vi "Get Build Version.vi"(8 "error in":errorcluster caption="Error In", 10 "Build Spec Name":string, 11 "Project Path":path) -> (0 "error out":errorcluster caption="Error Out", 3 "Version":string)   [LabVIEW 2015]
doc: "Open the VI reference pointed by the VI Name input. This function does not require a path as input but requires that the VI is present in the same project as the calling VI."
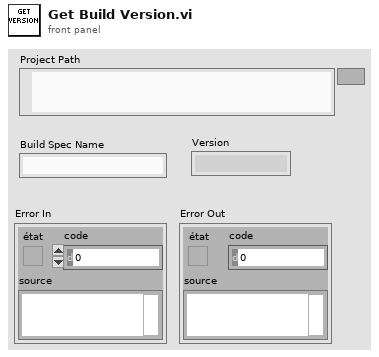
[diagram p1: front panel]
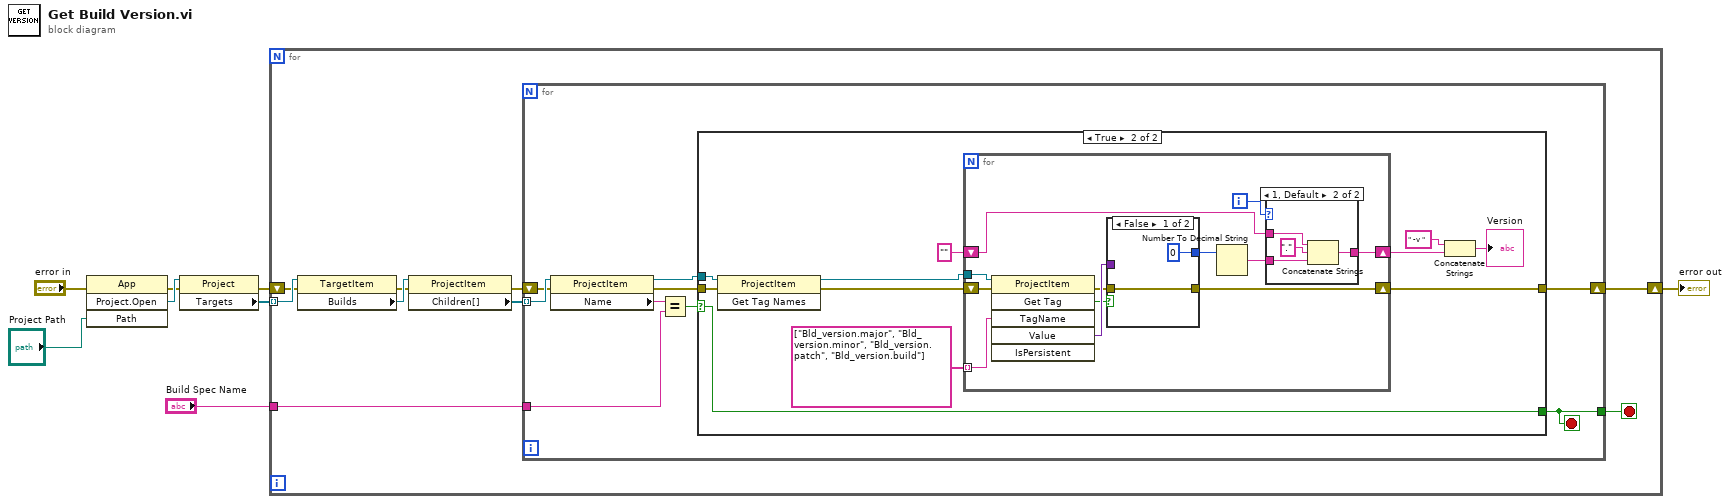
[diagram p0: block diagram]
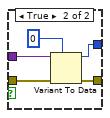
[diagram p4: hidden frame]
diagram:
  n1 = invoke class="App" method="Project.Open"(error in="error in", "Path"="Project Path") -> (error out=w4:errorcluster, "Project:Open"=w5:refnum<vi>)  [unwired: 2 in, 2 out]
  n2 = property class="Project"(reference=w5, error in=w4) -> (error out=w2:errorcluster, "Targets"=w8:refnum<vi>[])  [unwired: 1 out]
  n3 = for {
    tunnel: w8 -> [w17] mode=indexing
    tunnel: "Build Spec Name" -> [w14]
    shift-right: [w9] -> w1
    shift-left: w2 -> [w10]
    stop <- w12 stop-if-true
    n4 = property class="TargetItem"(reference=w17, error in=w10) -> (error out=w13:errorcluster, "Builds"=w16:refnum<vi>)  [unwired: 1 out]
    n5 = property class="ProjectItem"(reference=w16, error in=w13) -> (error out=w11:errorcluster, "Children[]"=w15:refnum<vi>[])  [unwired: 1 out]
    n6 = for {
      tunnel: w15 -> [w24] mode=indexing
      tunnel: w14 -> [w25]
      tunnel: [w22] -> w12
      shift-right: [w18] -> w9
      shift-left: w11 -> [w21]
      stop <- w22 stop-if-true
      n7 = property class="ProjectItem"(reference=w24, error in=w21) -> (reference out=w19:refnum<vi>, error out=w20:errorcluster, "Name"=w26:string)
      n8 = Equal?(x=w26, y=w25) -> (x = y?=w23:bool)
      n9 = case shown="True" w23 {
        selector: w23 -> [_ w37]
        tunnel: w19 -> [_ w38]
        tunnel: [_ w37] -> w22
        tunnel: w20 -> [w27 w33]
        tunnel: [w27 w31] -> w18
        frame False {
        }
        frame True {
          n10 = invoke class="ProjectItem" method="Get Tag Names"(reference=w38, error in=w33) -> (reference out=w36:refnum<vi>, error out=w32:errorcluster)  [unwired: 1 in, 1 out]
          n11 = for {
            tunnel: w36 -> [w49]
            tunnel: string[] ["Bld_version.major", "Bld_version.minor", "Bld_version.patch", "Bld_version.build"] -> [w48] mode=indexing
            shift-right: [w43] -> w29
            shift-left: "" -> [w44]
            shift-right: [w39] -> w31
            shift-left: w32 -> [w41]
            i -> [w42]
            n12 = invoke class="ProjectItem" method="Get Tag"(reference=w49, error in=w41, "TagName"=w48) -> (error out=w40:errorcluster, "GetTag"=w47:bool, "Value"=w50:variant)  [unwired: 3 in, 3 out]
            n13 = case shown="False" w47 {
              tunnel: w50 -> [_ w62]
              tunnel: [0 w60] -> w46
              tunnel: w40 -> [w56 w59]
              tunnel: [w56 w58] -> w39
              frame False {
              }
              frame True {
                n14 = Variant To Data(error in=w59, type=0, Variant=w62) -> (data=w60:i32, error out=w58:errorcluster)
              }
            }
            n15 = Number To Decimal String(number=w46) -> (decimal integer string=w45:string)  [unwired: 1 in]
            n16 = case shown="1, Default" w42 {
              tunnel: w45 -> [w51 w55]
              tunnel: w44 -> [_ w53]
              tunnel: [w51 w54] -> w43
              frame 0 {
              }
              frame 1, Default {
                n17 = Concatenate Strings(w53, "." ("string"), w55) -> (w54:string)
              }
            }
          }
          n18 = Concatenate Strings(" -v " ("string"), w29) -> (→"Version":string)
        }
      }
    }
  }
  "error out" <- w1
